vi "DSF.Shared.Configuration.Plugin.Initialize.vi"(4 "Priority":u8, 6 "Cycle Timing Factors":T1={"Decimation"=1, "Offset"=0}, 7 "Custom Parameters":variant, 8 "error in (no error)":errorcluster, 9 "Transfer Group Configurations":refnum<class "DSF.Shared.Configuration.Transfer Group.lvclass">[](array[class]), 10 "Name":string, 11 "Plugin Configuration in":refnum<class "DSF.Shared.Configuration.Plugin.lvclass">) -> (0 "error out":errorcluster, 3 "Plugin Configuration out":refnum<class "DSF.Shared.Configuration.Plugin.lvclass">)   [LabVIEW 2016, in "DSF.Shared.lvlib" / "DSF.Shared.Configuration.Plugin.lvclass"]
uses:
  DSF.Shared.Configuration.Plugin.lvclass
  C:/Git/SourceTree/DSF/Source/Shared/Classes/Configuration/DSF.Shared.Configuration.Cycle Timed.lvclass
  Typedefs/DSF.Shared.Typedefs.Cycle Timing Factors.ctl
  Transfer Group/DSF.Shared.Configuration.Transfer Group.lvclass
  DSF.Shared.Configuration.Plugin.lvclass/DSF.Shared.Configuration.Plugin.ctl
  Configuration/DSF.Shared.Configuration.Cycle Timed.lvclass
  DSF.Shared.lvlib
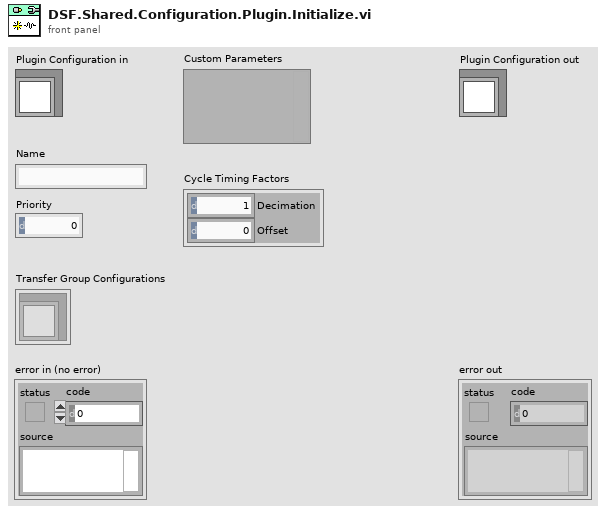
[diagram p1: front panel]
types:
  T1 = typedef "DSF.Shared.lvlib/DSF.Shared.Typedefs.Cycle Timing Factors.ctl" = cluster{"Decimation":u64, "Offset":u64}
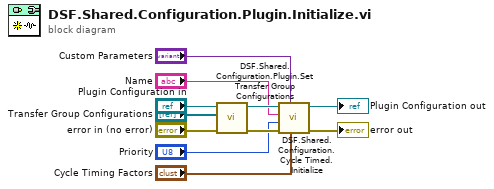
[diagram p0: block diagram]
diagram:
  n1 = call "DSF.Shared.Configuration.Plugin.Set Transfer Group Configurations.vi"("error in (no error)"="error in (no error)", "Transfer Group Configurations"="Transfer Group Configurations", "Plugin Configuration in"="Plugin Configuration in") -> ("error out"=w4:errorcluster, "Plugin Configuration out"=w5:refnum<class "DSF.Shared.Configuration.Plugin.lvclass">)  [unwired: 7 in]
  n2 = call "DSF.Shared.Configuration.Cycle Timed.Initialize.vi"("Cycle Timing Factors"="Cycle Timing Factors", "Custom Parameters"="Custom Parameters", "error in (no error)"=w4, "Priority"="Priority", "Name"="Name", "Cycle Timed Configuration in"=w5) -> ("error out"=→"error out":errorcluster, "Cycle Timed Configuration out"=→"Plugin Configuration out":refnum<class "DSF.Shared.Configuration.Plugin.lvclass">)  [unwired: 4 in]
